vi "core_s2ms.vi"(2 "s {DBL}":dbl format="%#_13g") -> (7 "ms {I32}":i32)   [LabVIEW 2015]
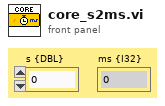
[diagram p1: front panel]
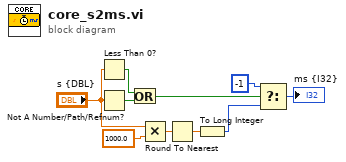
[diagram p0: block diagram]
diagram:
  n1 = Less Than 0?(x="s {DBL}") -> (x < 0?=w8:bool)
  n2 = Not A Number/Path/Refnum?(number/path/refnum="s {DBL}") -> (NaN/Path/Refnum?=w7:bool)
  n3 = Or(x=w8, y=w7) -> (x .or. y?=w6:bool)
  n4 = Multiply(x="s {DBL}", y=1000.0) -> (x*y=w5:dbl)
  n5 = Round To Nearest(number=w5) -> (nearest integer value=w4:dbl)
  n6 = To Long Integer(number=w4) -> (32bit integer=w2:i32)
  n7 = Select(t=-1 ("s? t:f"), s=w6, f=w2) -> (s? t:f=→"ms {I32}":i32)
